vi "scratch.vi"() -> ()   [LabVIEW 2015]
uses:
  rapidjson wrapper/jsonType.ctl
  API/JSON Document Class/json query/json Query - string path.vi
  API/JSON Document Class/json parse/poly instances/json Parse Double Array - string path.vi
  API/JSON Document Class/json insert/poly instances/json Insert Double Array - string path.vi
  API/JSON Document Class/json to string/json To Minimized String - string path.vi
  API/JSON Document Class/JSON Document.lvclass
  rapidjson wrapper/rapidjson wrapper.lvlib
panel:
  out "value":dbl[](array[numeric])
  out "defaulted indices":i32[](array[numeric])
  out "defaulted?":bool
  out "type":T1
  out "json string":string
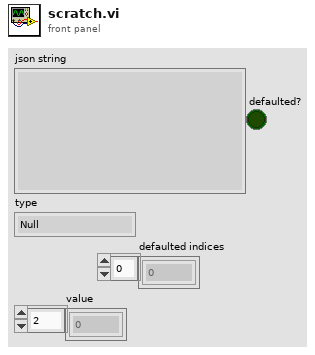
[diagram p1: front panel]
types:
  T1 = typedef "rapidjson wrapper.lvlib/jsonType.ctl" = enum16{"Null", "False", "True", "Object", "Array", "String", "Number"}
  T2 = cluster{"enable extensions?":bool, "allow comments?":bool}
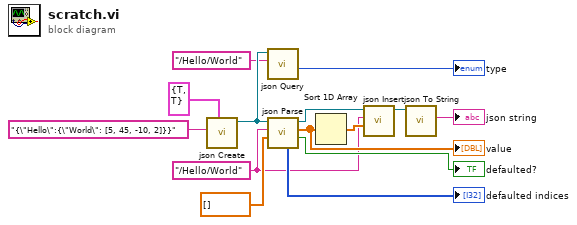
[diagram p0: block diagram]
diagram:
  w2 = "/Hello/World" ("path")
  n1 = call "json Create.vi"("options"=T2 {"enable extensions?"=TRUE, "allow comments?"=TRUE}, "JSON String"="{\"Hello\":{\"World\": [5, 45, -10, 2]}}") -> ("JSON Document out"=w11:refnum<class "JSON Document.lvclass">)  [unwired: 8 in, 1 out]
  n2 = call-poly "json Query.vi"("path"="/Hello/World", "JSON Document in"=w11) -> ("type"=→"type":T1)  [unwired: 6 in, 3 out]
  n3 = call-poly "json Parse.vi"("default"=dbl[] [], "path"=w2, "JSON Document in"=w11) -> ("defaulted?"=→"defaulted?":bool, "value"=w5:dbl[], "JSON Document out"=w4:refnum<class "JSON Document.lvclass">, "defaulted indices"=→"defaulted indices":i32[])  [unwired: 4 in, 1 out]
  "value" <- w5
  n4 = Sort 1D Array(array=w5) -> (sorted array=w3:dbl[])
  n5 = call-poly "json Insert.vi"("anything"=w3, "path"=w2, "JSON Document in"=w4) -> ("JSON Document out"=w1:refnum<class "JSON Document.lvclass">)  [unwired: 6 in, 2 out]
  n6 = call-poly "json To String.vi"("JSON Document in"=w1) -> ("json string"=→"json string":string)  [unwired: 8 in, 2 out]
